vi "run reference with parameters.vi"(7 "reentrant? (T)":bool=TRUE, 8 "error in":errorcluster, 9 "data":variant[](array[variant]), 10 "terminals":string[](array[string]), 11 "VI Refnum":refnum<vi>) -> (0 "error out":errorcluster)   [LabVIEW 2013, in "NISE Tools VI Server.lvlib"]
doc: "Runs a VI using the run VI method, providing it with any input parameters. This instance accepts a VI server refnum."
uses:
  NISE Tools VI Server.lvlib
  run VI with parameters.vi
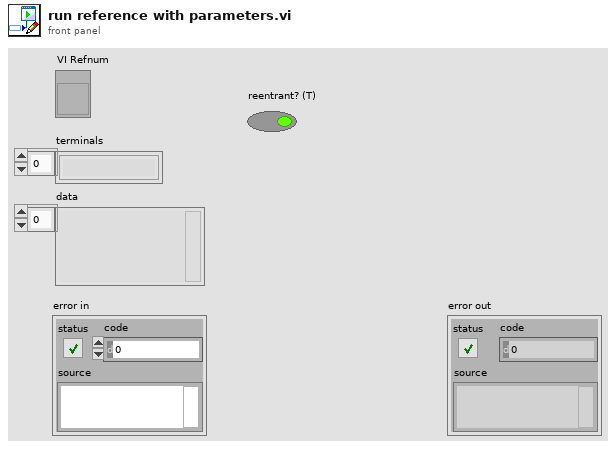
[diagram p1: front panel]
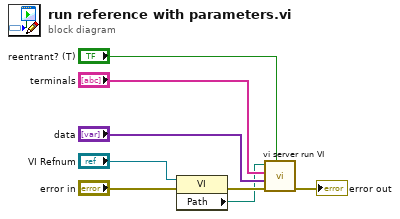
[diagram p0: block diagram]
diagram:
  n1 = property class="VI"(reference="VI Refnum", error in="error in") -> (error out=w6:errorcluster, "Path"=w3:path)  [unwired: 1 out]
  n2 = call-poly "vi server run VI.vi"("reentrant? (T)"="reentrant? (T)", "error in"=w6, "data"="data", "terminals"="terminals", "VI path"=w3) -> ("error out"=→"error out":errorcluster)  [unwired: 6 in]
